vi "SymmetricalCompoentsToO.vi"() -> ()   [LabVIEW 2015]
uses:
  AlphaBetaAndDQ_variants/AlphaBetaToDQ_src.vi
  <vilib>/addons/Electrical Power/Basic/NI_EP_Basic.lvlib
panel:
  out "inverse":sgl[][](graph)
  out "appended array":dbl[][](graph)
  in  "C_Mag":dbl format="%#_13g"
  in  "B_Mag":dbl format="%#_13g"
  in  "A_Mag":dbl format="%#_13g"
  out "waveforms":dbl[][](graph)
  in  "stop":bool
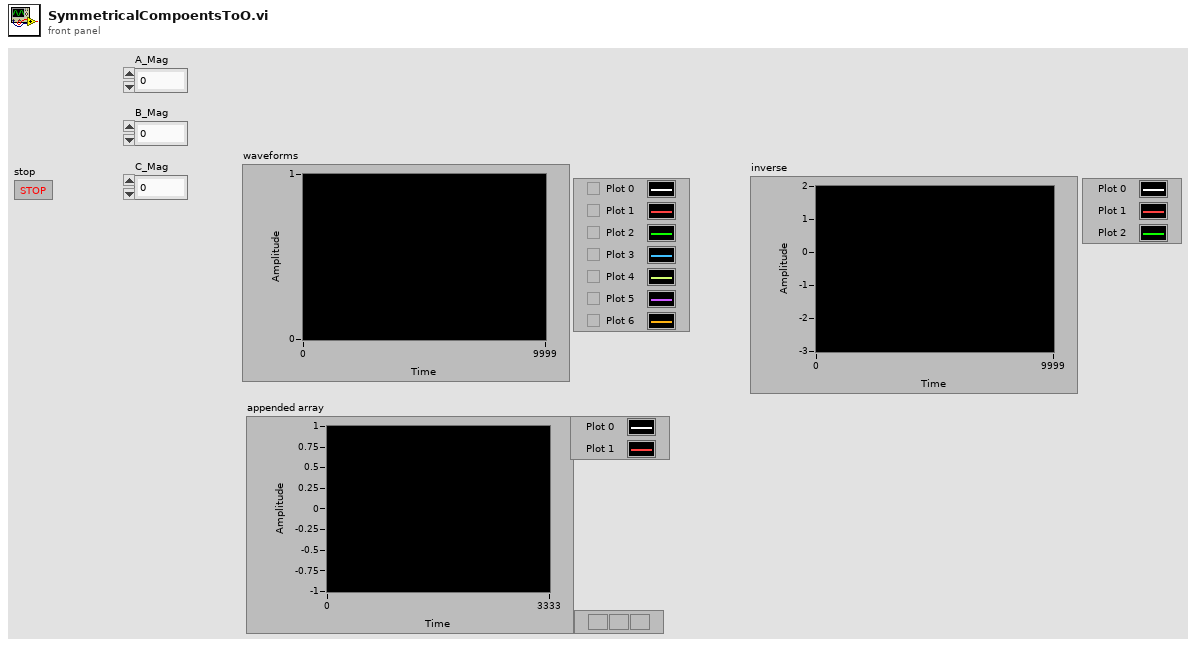
[diagram p1: front panel]
types:
  T1 = typedef "ComplexSGL" = cluster{"real":sgl, "img":sgl}
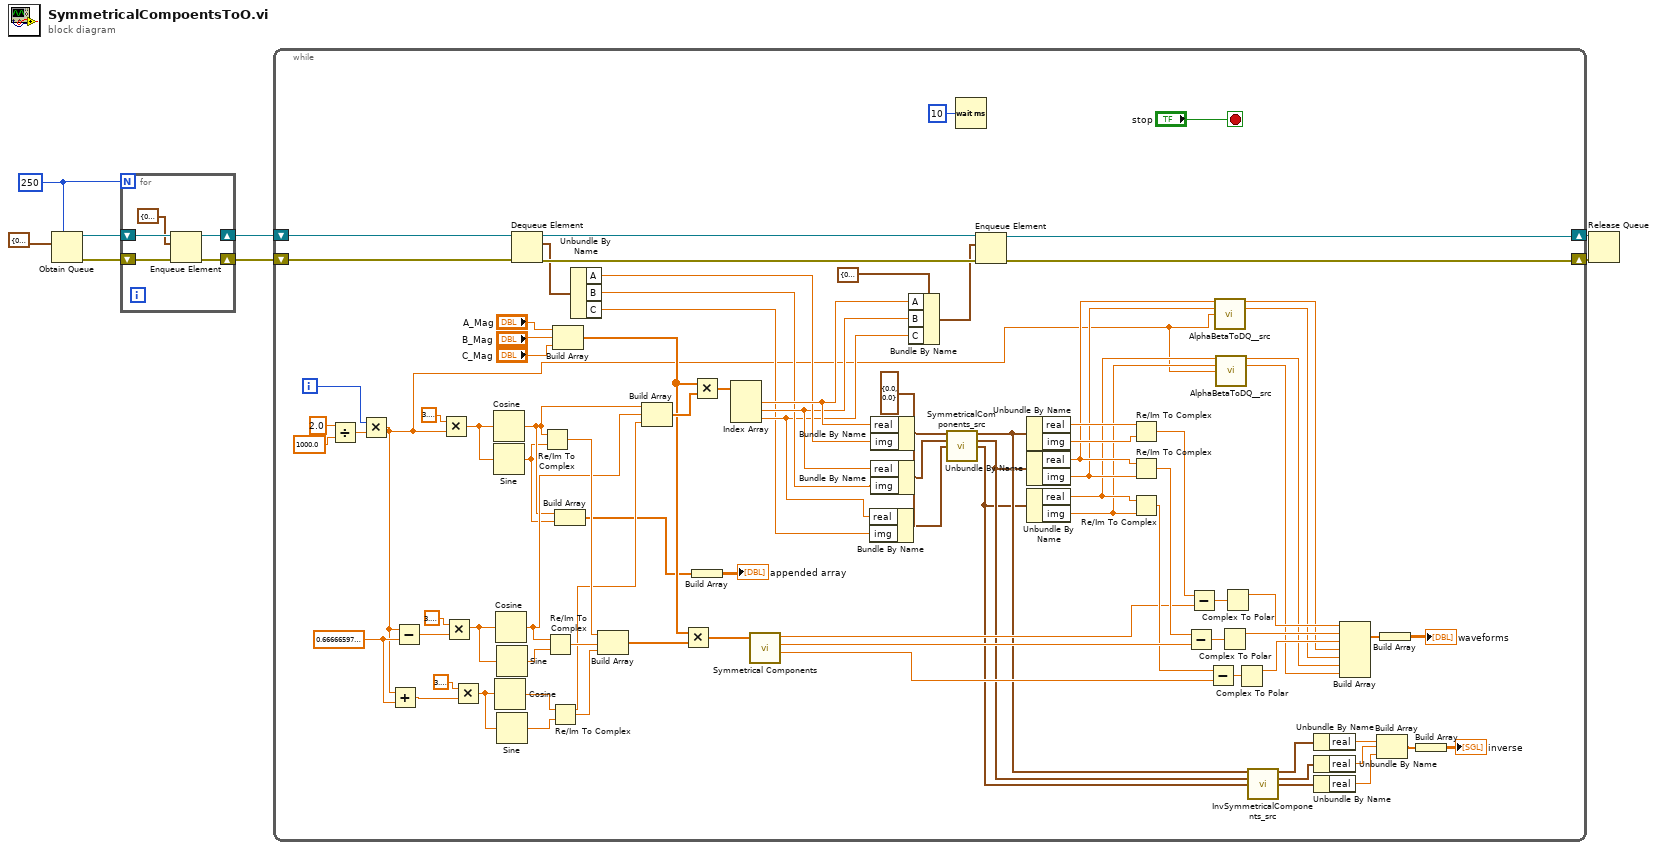
[diagram p0: block diagram]
diagram:
  w1 = 250 ("max queue size (-1, unlimited)")
  n1 = Obtain Queue(max queue size (-1, unlimited)=w1, element data type=cluster{"A":dbl, "B":dbl, "C":dbl} {"A"=0.0, "B"=0.0, "C"=0.0}) -> (queue out=w7:refnum<queue>, error out=w6:errorcluster)  [unwired: 3 in, 1 out]
  n2 = for {
    N: w1 -> [_]
    shift-right: [w11] -> w5
    shift-left: w7 -> [w13]
    shift-right: [w10] -> w4
    shift-left: w6 -> [w12]
    n3 = Enqueue Element(queue=w13, element=cluster{"A":dbl, "B":dbl, "C":dbl} {"A"=0.0, "B"=0.0, "C"=0.0}, error in (no error)=w12) -> (queue out=w11:refnum<queue>, error out=w10:errorcluster)  [unwired: 1 in, 1 out]
  }
  n4 = while {
    shift-right: [w86] -> w3
    shift-left: w4 -> [w90]
    shift-right: [w87] -> w2
    shift-left: w5 -> [w91]
    i -> [w93]
    stop <- "stop" stop-if-true
    w58 = T1 {"real"=0.0, "img"=0.0} ("A")
    w101 = sgl 0.666666 ("y")
    n5 = Divide(x=sgl 2.0, y=sgl 1000.0) -> (x/y=w92:sgl)
    n6 = Multiply(x=w93, y=w92) -> (x*y=w29:sgl)
    n7 = Add(x=w29, y=w101) -> (x+y=w96:sgl)
    n8 = Subtract(x=w29, y=w101) -> (x-y=w100:sgl)
    n9 = Multiply(x=3.141592653589793, y=w29) -> (x*y=w34:dbl)
    n10 = Multiply(x=3.141592653589793, y=w100) -> (x*y=w81:dbl)
    n11 = Multiply(x=3.141592653589793, y=w96) -> (x*y=w82:dbl)
    n12 = Cosine(x=w34) -> (cos(x)=w28:dbl)
    n13 = Sine(x=w34) -> (sin(x)=w27:dbl)
    n14 = Cosine(x=w82) -> (cos(x)=w73:dbl)
    n15 = Cosine(x=w81) -> (cos(x)=w74:dbl)
    n16 = Sine(x=w81) -> (sin(x)=w80:dbl)
    n17 = Sine(x=w82) -> (sin(x)=w79:dbl)
    n18 = Dequeue Element(queue=w91, error in (no error)=w90) -> (queue out=w89:refnum<queue>, element=w85:cluster{"A":dbl, "B":dbl, "C":dbl}, error out=w88:errorcluster)  [unwired: 1 in, 1 out]
    n19 = Re/Im To Complex(1:w27, 2:w28) -> (0:w77:cdb)
    n20 = Re/Im To Complex(1:w80, 2:w74) -> (0:w78:cdb)
    n21 = Re/Im To Complex(1:w79, 2:w73) -> (0:w76:cdb)
    n22 = Build Array("A_Mag", "B_Mag", "C_Mag") -> (w41:dbl[])
    n23 = Build Array(w28, w27) -> (w26:dbl[])
    n24 = Unbundle By Name(w85) -> ("A"=w59:dbl, "B"=w56:dbl, "C"=w54:dbl)
    n25 = Build Array(w77, w78, w76) -> (w71:cdb[])
    n26 = Build Array(w28, w74, w73) -> (w72:dbl[])
    n27 = Multiply(x=w41, y=w71) -> (x*y=w70:cdb[])
    n28 = Multiply(x=w41, y=w72) -> (x*y=w69:dbl[])
    n29 = Build Array(w26) -> (→"appended array":dbl[][])
    n30 = Index Array(array=w69) -> (element #1=w60:dbl, element #2=w57:dbl, element #3=w55:dbl)  [unwired: 3 in]
    n31 = call <vilib>:"Symmetrical Components.vi"("3-phase phasors"=w70) -> ("negative sequence"=w67:cdb, "positive sequence"=w68:cdb, "zero sequence"=w47:cdb)  [unwired: 7 in, 1 out]
    n32 = Bundle By Name(cluster=w58, "real"=w55, "img"=w54) -> (w51:T1)
    n33 = Bundle By Name(cluster=w58, "real"=w60, "img"=w59) -> (w53:T1)
    n34 = Bundle By Name(cluster=w58, "real"=w57, "img"=w56) -> (w52:T1)
    n35 = Bundle By Name(cluster=cluster{"A":dbl, "B":dbl, "C":dbl} {"A"=0.0, "B"=0.0, "C"=0.0}, "A"=w60, "B"=w57, "C"=w55) -> (w84:cluster{"A":dbl, "B":dbl, "C":dbl})
    n36 = call "SymmetricalComponents_src.vi"("A"=w53, "B"=w52, "C"=w51) -> ("zero"=w24:T1, "positive"=w23:T1, "negative"=w22:T1)  [unwired: 10 in]
    n37 = Wait (ms)(milliseconds to wait=u32 10) -> ()  [unwired: 1 out]
    n38 = Enqueue Element(queue=w89, element=w84, error in (no error)=w88) -> (queue out=w87:refnum<queue>, error out=w86:errorcluster)  [unwired: 1 in, 1 out]
    n39 = Unbundle By Name(w24) -> ("real"=w40:sgl, "img"=w39:sgl)
    n40 = Unbundle By Name(w23) -> ("real"=w38:sgl, "img"=w37:sgl)
    n41 = Unbundle By Name(w22) -> ("real"=w36:sgl, "img"=w35:sgl)
    n42 = Re/Im To Complex(1:w39, 2:w40) -> (0:w46:csg)
    n43 = Re/Im To Complex(1:w37, 2:w38) -> (0:w50:csg)
    n44 = Re/Im To Complex(1:w35, 2:w36) -> (0:w49:csg)
    n45 = Subtract(x=w50, y=w68) -> (x-y=w66:cdb)
    n46 = Subtract(x=w46, y=w47) -> (x-y=w48:cdb)
    n47 = Subtract(x=w49, y=w67) -> (x-y=w64:cdb)
    n48 = call-poly "AlphaBetaToDQ__src.vi"("alpha"=w38, "beta"=w37, "theta"=w29) -> ("direct"=w33:sgl, "quadrature"=w32:sgl)  [unwired: 9 in, 2 out]
    n49 = call-poly "AlphaBetaToDQ__src.vi"("alpha"=w36, "beta"=w35, "theta"=w29) -> ("direct"=w31:sgl, "quadrature"=w30:sgl)  [unwired: 9 in, 2 out]
    n50 = Complex To Polar(r * e^(i*theta)=w66) -> (r=w65:dbl)  [unwired: 1 out]
    n51 = Complex To Polar(r * e^(i*theta)=w48) -> (r=w45:dbl)  [unwired: 1 out]
    n52 = Complex To Polar(r * e^(i*theta)=w64) -> (r=w63:dbl)  [unwired: 1 out]
    n53 = call "InvSymmetricalComponents_src.vi"("zero"=w24, "positive"=w23, "negative"=w22) -> ("a"=w21:T1, "b"=w19:T1, "c"=w20:T1)  [unwired: 10 in]
    n54 = Unbundle By Name(w21) -> ("real"=w18:sgl)
    n55 = Unbundle By Name(w19) -> ("real"=w17:sgl)
    n56 = Unbundle By Name(w20) -> ("real"=w16:sgl)
    n57 = Build Array(w45, w65, w63, w33, w32, w31, w30) -> (w62:dbl[])
    n58 = Build Array(w18, w17, w16) -> (w15:sgl[])
    n59 = Build Array(w62) -> (→"waveforms":dbl[][])
    n60 = Build Array(w15) -> (→"inverse":sgl[][])
  }
  n61 = Release Queue(queue=w2, error in (no error)=w3) -> ()  [unwired: 1 in, 3 out]
